vi "teste_1.vi"() -> ()   [LabVIEW 2025]
panel:
  out "Farenheit":dbl
  in  "Celsius":dbl
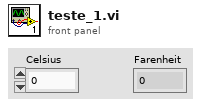
[diagram p1: front panel]
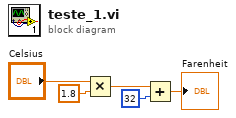
[diagram p0: block diagram]
diagram:
  n1 = Multiply(x="Celsius", y=1.8) -> (x*y=w2:dbl)
  n2 = Add(x=w2, y=32) -> (x+y=→"Farenheit":dbl)
